vi "GetAllProperties.vi"(8 "error in (no error)":errorcluster, 11 "CSSProperties in":refnum<class "CSSProperties.lvclass">) -> (0 "error out":errorcluster, 2 "Properties":string[](array[string]), 3 "CSSProperties out":refnum<class "CSSProperties.lvclass">)   [LabVIEW 2019, in "CSSProperties.lvclass"]
uses:
  CSSProperties.lvclass
  CSSProperties.lvclass/CSSProperties.ctl
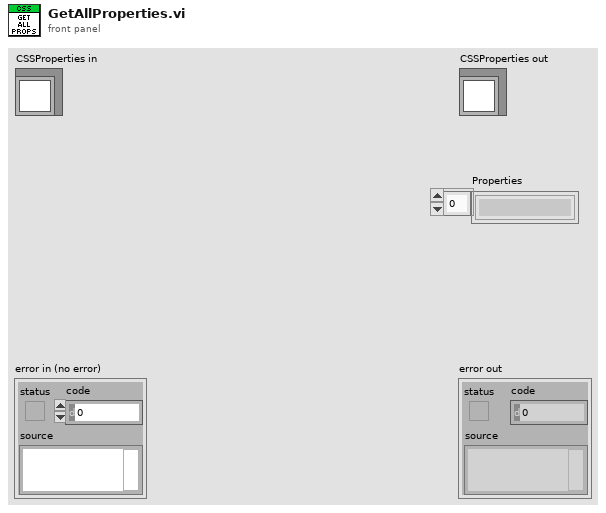
[diagram p1: front panel]
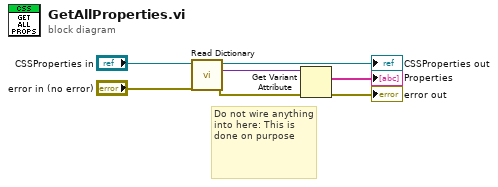
[diagram p0: block diagram]
diagram:
  # "Do not wire anything into here: This is done on purpose"
  n1 = call "Read Dictionary.vi"("error in (no error)"="error in (no error)", "CSSProperties in"="CSSProperties in") -> ("error out"=w4:errorcluster, "Dictionary"=w7:variant, "CSSProperties out"=→"CSSProperties out":refnum<class "CSSProperties.lvclass">)  [unwired: 7 in]
  n2 = Get Variant Attribute(Variant=w7, error in=w4) -> (names=→"Properties":string[], error out=→"error out":errorcluster)  [unwired: 2 in, 2 out]
